vi "append_to_log.vi"(5 "data_type":T1, 7 "dims":T2, 8 "error in (no error)":errorcluster, 9 "Location":string, 10 "Data":variant, 11 "scan_hdf5_log in":refnum<class "scan_2d_hdf5_log.lvclass">) -> (0 "error out":errorcluster, 3 "scan_hdf5_log out":refnum<class "scan_2d_hdf5_log.lvclass">)   [LabVIEW 2015, in "scan_2d_hdf5_log.lvclass"]
uses:
  scan_2d_hdf5_log.lvclass
  Data Logger Class/data_dimensionality.ctl
  Data Logger Class/logger_data_types.ctl
  detector_data_tdef.ctl
  scan_2d_hdf5_log.lvclass/scan_2d_hdf5_log.ctl
  <vilib>/Utility/miscctls.llb/LVRectTypeDef.ctl
  <vilib>/UPVI/lvhdf5/group.llb/H5G_obj_t.ctl
  <vilib>/UPVI/lvhdf5/dataset.llb/LVH5D Operation.ctl
  <vilib>/UPVI/lvhdf5/utility.llb/Select HDF5 Dialog.vi
  <vilib>/UPVI/lvhdf5/utility.llb/Select HDF5 Dialog (Object Only).vi
  <vilib>/UPVI/lvhdf5/dataset.llb/Simple H5Dwrite (Variant).vi
  <vilib>/UPVI/lvhdf5/dataset.llb/Simple H5Dwrite.xnode
  <vilib>/UPVI/lvhdf5/library.llb/HDF5 Ref.ctl
  <vilib>/UPVI/lvhdf5/file.llb/H5Fclose.vi
  <vilib>/UPVI/lvhdf5/identifier.llb/Not an HDF5 Refnum Constant.vi
  <vilib>/Utility/error.llb/Error Cluster From Error Code.vi
  <vilib>/UPVI/lvhdf5/dataset.llb/OpenCreateReplace Dataset by Element Type.vi
  <vilib>/UPVI/lvhdf5/dataspace.llb/H5Sselect_hyperslab.vi
  <vilib>/UPVI/lvhdf5/dataset.llb/H5Dwrite (Variant).vi
  <vilib>/UPVI/lvhdf5/dataset.llb/H5Dget_space.vi
  <vilib>/UPVI/lvhdf5/attribute.llb/private/LVH5AwriteWDTAttrs.vi
  <vilib>/UPVI/lvhdf5/dataspace.llb/H5Sclose.vi
  <vilib>/UPVI/lvhdf5/file.llb/OpenCreateReplace HDF5 File.vi
  <vilib>/UPVI/lvhdf5/file.llb/LVH5F Operation.ctl
  <vilib>/UPVI/lvhdf5/utility.llb/Select HDF5 Dialog (File and Object).vi
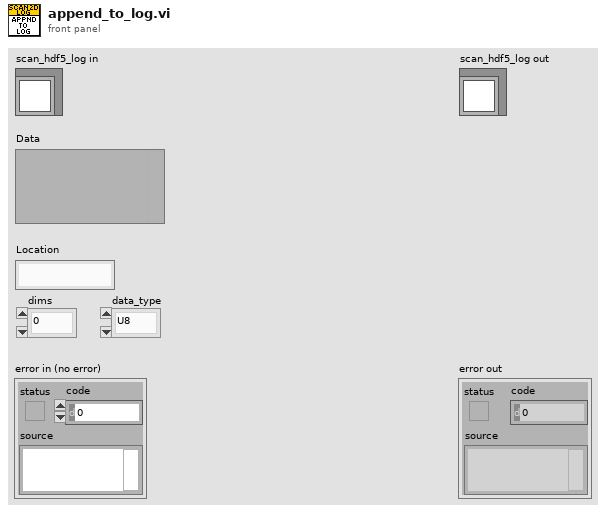
[diagram p1: front panel]
types:
  T1 = typedef "logger_data_types.ctl" = enum16{"U8", "I8", "U16", "I16", "U32", "I32", "DBL", "String"}
  T2 = typedef "data_dimensionality.ctl" = enum16{"0", "1", "2"}
  T3 = typedef "detector_data_tdef.ctl" = cluster{"data_array":dbl[][][], "data_size":cluster{"X":i32, "Y":i32, "Z":i32}}
  T4 = typedef "LVRectTypeDef.ctl" = cluster{"Left":i16, "Top":i16, "Right":i16, "Bottom":i16}
  T5 = cluster{"Behavior":enum32{"Invalid", "Default", "Floating", "Floating/Auto-Hide", "Modal"}, "Position":T4, "Center":bool, "Title":string}
  T6 = typedef "LVH5F Operation.ctl" = enum16{"open", "open or create", "create or replace", "create or replace (with confirmation)", "create", "open (read only)"}
  T7 = typedef "LVH5D Operation.ctl" = enum16{"open", "replace", "create", "open or create", "create or replace", "create or replace with confirmation"}
  T8 = typedef "H5G_obj_t.ctl" = i32
  T9 = cluster{"Object Types (any)":T8[], "Object Pattern":string}
  T10 = typedef "HDF5 Ref.ctl" = refnum<k1>
  T11 = typedef "data_types_tdef.ctl" = enum16{"0D", "1D", "2D"}
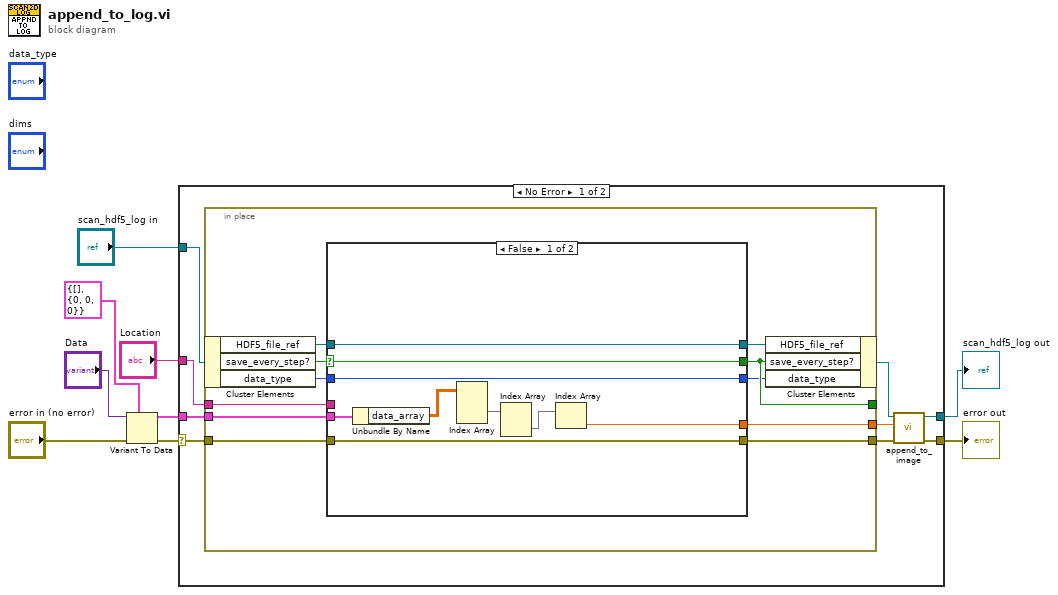
[diagram p0: block diagram]
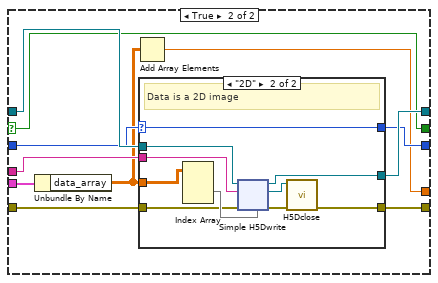
[diagram p2: hidden frame]
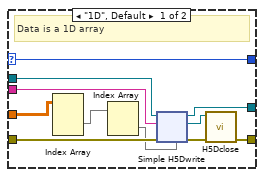
[diagram p3: hidden frame]
diagram:
  n1 = Variant To Data(error in="error in (no error)", type=T3 {"data_array"=[], "data_size"={"X"=0, "Y"=0, "Z"=0}} ("image_data"), Variant="Data") -> (data=w8:T3, error out=w3:errorcluster)
  n2 = case shown="No Error" w3 {
    selector: w3 -> [w15 w475]
    tunnel: w8 -> [w18 _]
    tunnel: "scan_hdf5_log in" -> [w17 w476]
    tunnel: "Location" -> [w16 _]
    tunnel: [w13 w475] -> w2
    tunnel: [w11 w476] -> w1
    frame No Error {
      n3 = in-place {
        in-place-border: w18 -> [w29]
        in-place-border: w16 -> [w24]
        in-place-border: w15 -> [w26]
        in-place-border: [w25] -> w14
        in-place-border: [w21] -> w10
        in-place-border: [w20] -> _
        n4 = in-place-cluster #1(w17) -> ("HDF5_file_ref"=w28:T10, "save_every_step?"=w22:bool, "data_type"=w23:T11)
        n5 = case shown="False" w22 {
          selector: w22 -> [w33 w41]
          tunnel: w29 -> [w38 w49]
          tunnel: w28 -> [w31 w48]
          tunnel: [w31 w47] -> w27
          tunnel: w26 -> [w30 w46]
          tunnel: [w30 w45] -> w25
          tunnel: w24 -> [_ w44]
          tunnel: w23 -> [w32 w43]
          tunnel: [w34 w40] -> w21
          tunnel: [w33 w41] -> w20
          tunnel: [w32 w42] -> w19
          frame False {
            n6 = Unbundle By Name(w38) -> ("data_array"=w37:dbl[][][])
            n7 = Index Array(array=w37) -> (element=w36:dbl[][])  [unwired: 3 in]
            n8 = Index Array(array=w36) -> (element=w35:dbl[])  [unwired: 2 in]
            n9 = Index Array(array=w35) -> (element=w34:dbl)  [unwired: 1 in]
          }
          frame True {
            n10 = Unbundle By Name(w49) -> ("data_array"=w39:dbl[][][])
            n11 = Add Array Elements(numeric array=w39) -> (sum=w40:dbl)
            n12 = case shown="\"2D\"" w43 {
              selector: w43 -> [w50 w263]
              tunnel: w39 -> [w60 w272]
              tunnel: w48 -> [w57 w268]
              tunnel: [w56 w267] -> w47
              tunnel: w46 -> [w55 w266]
              tunnel: [w54 w265] -> w45
              tunnel: w44 -> [w53 w264]
              tunnel: [w50 w263] -> w42
              frame "1D", Default {
                # "Data is a 1D array"
                n13 = Index Array(array=w60) -> (element=w52:dbl[][])  [unwired: 3 in]
                n14 = Index Array(array=w52) -> (element=w51:dbl[])  [unwired: 2 in]
                n15 = xnode "Simple H5Dwrite"("Dataset Path"=w53, "error in (no error)"=w55, "HDF5 Path or Ref"=w57, "Data"=w51) -> ("HDF5 Dataset Ref out"=w59:T10, "HDF5 Ref out"=w56:T10, "error out"=w58:errorcluster)  [unwired: 4 in]
                n16 = call <vilib>:"H5Dclose.vi"("error in (no error)"=w58, "HDF5 Dataset Ref"=w59) -> ("error out"=w54:errorcluster)  [unwired: 7 in]
              }
              frame "2D" {
                # "Data is a 2D image"
                n17 = Index Array(array=w272) -> (element=w269:dbl[][])  [unwired: 3 in]
                n18 = xnode "Simple H5Dwrite"("Dataset Path"=w264, "error in (no error)"=w266, "HDF5 Path or Ref"=w268, "Data"=w269) -> ("HDF5 Dataset Ref out"=w271:T10, "HDF5 Ref out"=w267:T10, "error out"=w270:errorcluster)  [unwired: 4 in]
                n19 = call <vilib>:"H5Dclose.vi"("error in (no error)"=w270, "HDF5 Dataset Ref"=w271) -> ("error out"=w265:errorcluster)  [unwired: 7 in]
              }
            }
          }
        }
        n20 = in-place-cluster #1("HDF5_file_ref"=w27, "save_every_step?"=w20, "data_type"=w19) -> (w12:refnum<class "scan_2d_hdf5_log.lvclass">)
      }
      n21 = call "append_to_image.vi"("error in (no error)"=w14, "data"=w10, "scan_2d_hdf5_log in"=w12) -> ("error out"=w13:errorcluster, "scan_2d_hdf5_log out"=w11:refnum<class "scan_2d_hdf5_log.lvclass">)  [unwired: 7 in]
    }
    frame Error {
    }
  }
  "error out" <- w2
  "scan_hdf5_log out" <- w1
